vi "WPs and Obstacles 3.vi"(11 "Real/Sim":bool) -> (0 "Obstacle Lats and Longs":cluster{"Obs Lats":dbl[], "Obs Longs":dbl[]} {"Obs Longs" format="%#_8g"; "Obs Lats" format="%#_8g"}, 1 "WP Lats and Longs":cluster{"WP Lats":dbl[], "WP Longs":dbl[]} {"WP Longs" format="%#_8g"; "WP Lats" format="%#_8g"}, 3 "WP Map":T1(graph))   [LabVIEW 2014]
panel:
  in  "Obstacle Real Longs":dbl[](array[numeric])=[81.2678, 81.267312, 81.267112, 81.267332, 81.267916, 81.267137, 81.267874, 81.267301, 81.267913, 81.26772] format="%#_8g"
  in  "Obstacle Real Lats":dbl[](array[numeric])=[37.1524, 37.152256, 37.152877, 37.152903, 37.152565, 37.152792, 37.152806, 37.152779, 37.152868, 37.152484] format="%#_8g"
  in  "WP Real Longs":dbl[](array[numeric])=[83.1954638, 83.19550076, 81.267112, 81.267332, 81.267916, 81.267137, 81.267874, 81.267301, 81.267913, 81.26772] format="%#_8g"
  in  "WP Real Lats":dbl[](array[numeric])=[42.678172477, 42.677950947, 37.152877, 37.152903, 37.152565, 37.152792, 37.152806, 37.152779, 37.152868, 37.152484] format="%#_8g"
  in  "WP Sim Longs":dbl[](array[numeric])=[81.267743, 81.267312, 81.267112, 81.267332, 81.267916, 81.267137, 81.267874, 81.267301, 81.267913, 81.26772] format="%#_8g"
  in  "WP Sim Lats":dbl[](array[numeric])=[37.152345, 37.152256, 37.152877, 37.152903, 37.152565, 37.152792, 37.152806, 37.152779, 37.152868, 37.152484] format="%#_8g"
  # "Waypoint and Obstacles 3 (Uses Paint)"
  # "20"
  # "12"
  # "Outputs:"
  # "Input:"
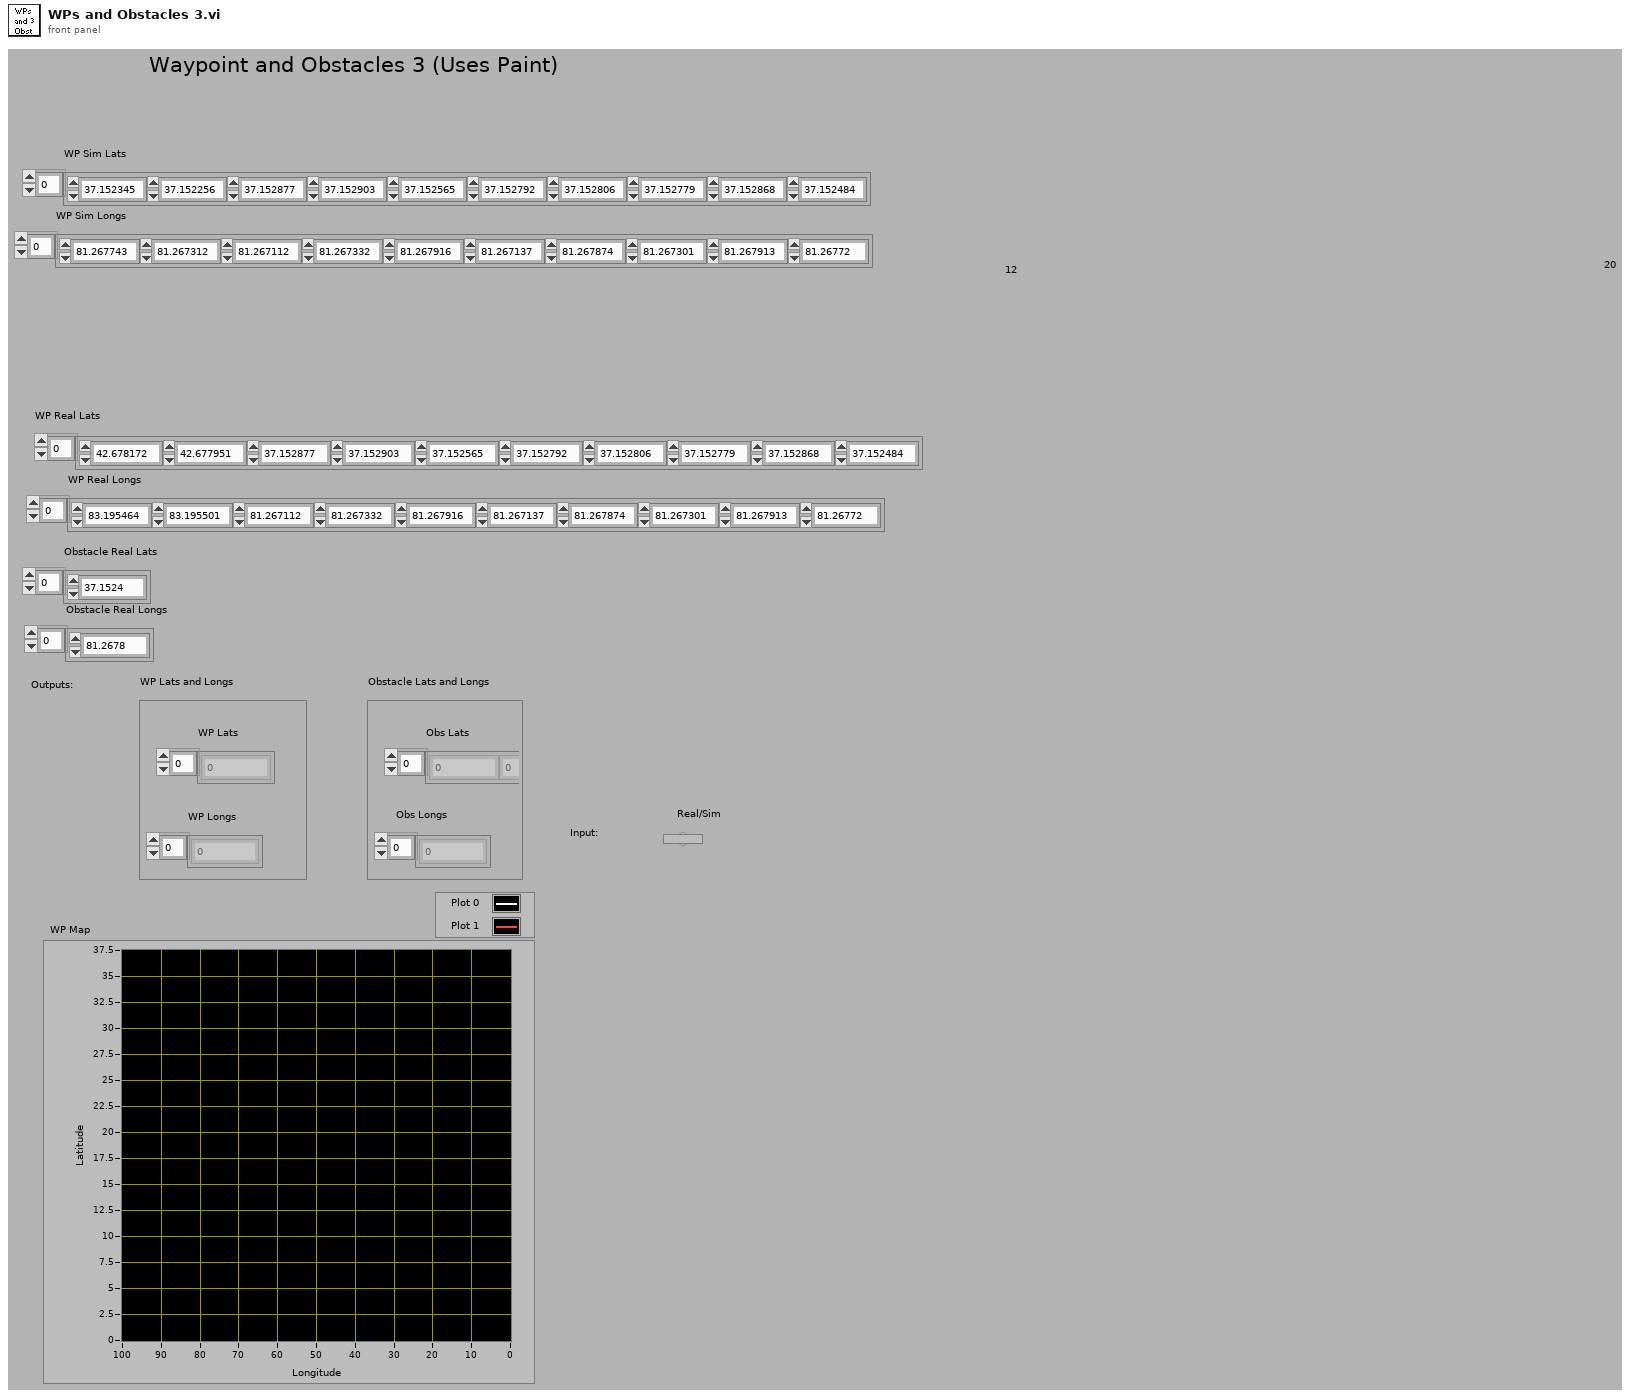
[diagram p1: front panel]
types:
  T1 = cluster{"Obstacle Longs":dbl[], "Obstacle Lats":dbl[]}[]
  T2 = cluster{"WP Sim Lats":dbl[], "WP Sim Longs":dbl[]}
  T3 = cluster{"Obstacle Longs":dbl[], "Obstacle Lats":dbl[]}
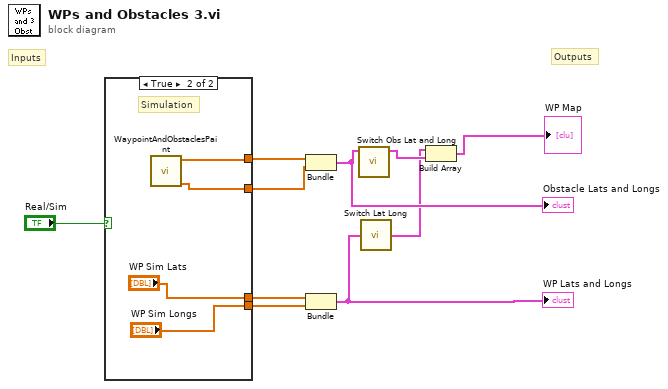
[diagram p0: block diagram]
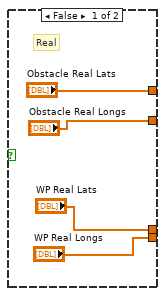
[diagram p2: hidden frame]
diagram:
  # "Inputs"
  # "Outputs"
  n1 = case shown="True" "Real/Sim" {
    tunnel: ["Obstacle Real Lats" w16] -> w9
    tunnel: ["Obstacle Real Longs" w15] -> w8
    tunnel: ["WP Real Lats" "WP Sim Lats"] -> w7
    tunnel: ["WP Real Longs" "WP Sim Longs"] -> w6
    frame False {
      # "Real"
    }
    frame True {
      # "Simulation"
      n2 = call "WaypointAndObstaclesPaint.vi"() -> ("Obs longs"=w15:dbl[], "Obs Lats"=w16:dbl[])  [unwired: 10 in]
    }
  }
  n3 = Bundle("Obs Lats"=w9, "Obs longs"=w8) -> (w4:cluster{"Obs Lats":dbl[], "Obs longs":dbl[]})  [unwired: 1 in]
  "Obstacle Lats and Longs" <- w4
  n4 = Bundle("WP Sim Lats"=w7, "WP Sim Longs"=w6) -> (w10:T2)  [unwired: 1 in]
  "WP Lats and Longs" <- w10
  n5 = call "Switch Obs Lat and Long.vi"("Obstacle Lats and Longs for GIC"=w4) -> ("Obstacle Lats and Longs switched"=w3:T3)  [unwired: 10 in]
  n6 = call "Switch Lat Long.vi"("WP Lats and Longs for GIC"=w10) -> ("WP Lats and Longs switched"=w2:cluster{"WP Longs":dbl[], "WP Lats":dbl[]})
  n7 = Build Array(w2, w3) -> (→"WP Map":T1)
